vi "Phase Correction.vi"(8 "error in (no error)":errorcluster, 9 "Y":dbl[](array[numeric]), 10 "X":dbl[](array[numeric]), 11 "Lockin Digitizer Driver in":refnum<class "Lockin Digitizer Driver.lvclass">) -> (0 "error out":errorcluster, 1 "Y out":dbl[](array[numeric]), 2 "X out":dbl[](array[numeric]), 3 "Lockin Digitizer Driver out":refnum<class "Lockin Digitizer Driver.lvclass">)   [LabVIEW 2021, in "Lockin Digitizer Driver.lvclass"]
uses:
  Lockin Digitizer Driver.lvclass
  Lockin Digitizer Driver.lvclass/Lockin Digitizer Driver.ctl
  8c7c85df-dbe1-4be7-af7e-5f87645200bc.vi
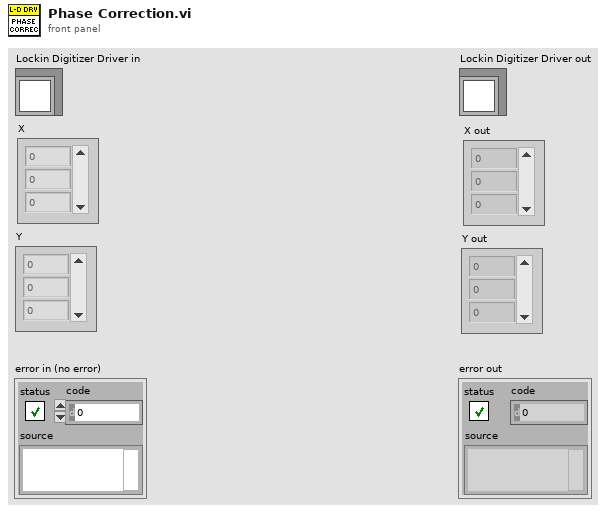
[diagram p1: front panel]
types:
  T1 = typedef "Lockin Digitizer Configuration.ctl" = cluster{"Post-trigger delay":dbl, "Post-trigger duration":dbl, "Rate":dbl, "Ranges":dbl[], "Re-name channels":string[], "Active channels":string, "External\nclock":bool, "Frequencies":dbl[], "Monitor time\nconstant":dbl, "Output \namplitudes":dbl[], "Input\nchannles":string[], "Sync":bool, "Lock-in input channel phases":dbl[]}
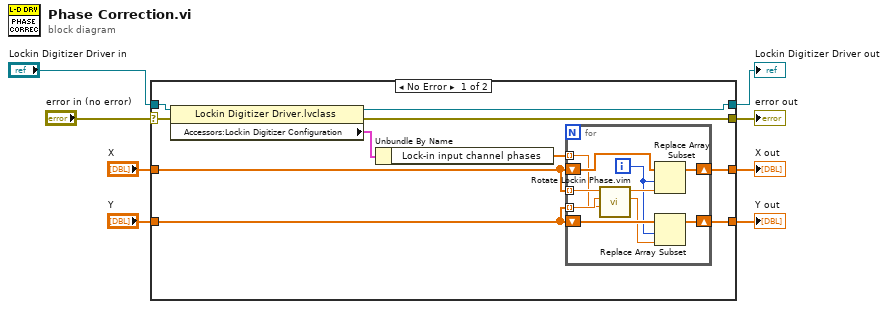
[diagram p0: block diagram]
diagram:
  n1 = case shown="No Error" "error in (no error)" {
    selector: "error in (no error)" -> [w18 w32]
    tunnel: [w17 w32] -> w7
    tunnel: [w15 w31] -> w5
    tunnel: "Lockin Digitizer Driver in" -> [w16 w31]
    tunnel: "X" -> [w12 w30]
    tunnel: "Y" -> [w11 w29]
    tunnel: [w10 w30] -> w2
    tunnel: [w9 w29] -> w1
    frame No Error {
      n2 = property class="Lockin Digitizer Driver.lvclass"(reference=w16, error in=w18) -> (reference out=w15:refnum<class "Lockin Digitizer Driver.lvclass">, error out=w17:errorcluster, "Accessors:Lockin Digitizer Configuration"=w14:T1)
      n3 = Unbundle By Name(w14) -> ("Lock-in input channel phases"=w13:dbl[])
      n4 = for {
        tunnel: w13 -> [w25] mode=indexing
        tunnel: w12 -> [w27] mode=indexing
        tunnel: w11 -> [w26] mode=indexing
        shift-right: [w23] -> w10
        shift-left: w12 -> [w28]
        shift-right: [w21] -> w9
        shift-left: w11 -> [w22]
        i -> [w19]
        n5 = call "Rotate Lockin Phase.vim"("Phase"=w25, "Array Y in"=w26, "Array X in"=w27) -> ("Array Y out"=w20:dbl, "Array X out"=w24:dbl)  [unwired: 7 in]
        n6 = Replace Array Subset(array=w28, new element=w24, index=w19) -> (w23:dbl[])
        n7 = Replace Array Subset(array=w22, new element=w20, index=w19) -> (w21:dbl[])
      }
    }
    frame Error {
    }
  }
  "error out" <- w7
  "Lockin Digitizer Driver out" <- w5
  "Y out" <- w1
  "X out" <- w2
